vi "Home.vi"() -> ()   [LabVIEW 2020]
doc: "Fonction :\n\nCe modèle peut être intégré très facilement à un subpannel à l'aide des fonctions de la palette Code Template >> Dynamic VI and Subpanel de la VIBOX"
uses:
  System.Windows.Forms
  <vilib>/Platform/TimedLoop/XDataNode/timing_clust.ctl
  <vilib>/Platform/TimedLoop/XDataNode/nitl_modes.ctl
  <vilib>/Platform/TimedLoop/XDataNode/wakeup.ctl
  <vilib>/Platform/TimedLoop/XDataNode/XDataNode.xnode
  Program Files (x86)/National Instruments/LabVIEW 2020/examples/DataGrid for LabVIEW/DataGrid.lvlib
  <vilib>/Platform/TimedLoop/XDataNode/XDNodeRunTimeDep.lvlib
panel:
  in  "今日计划":refnum<k24>(container)
  out "Stop<user event>":refnum<user-event>
  in  "当前生产统计":refnum<k24>(container)
  in  "当前生产状态":refnum<k24>(container)
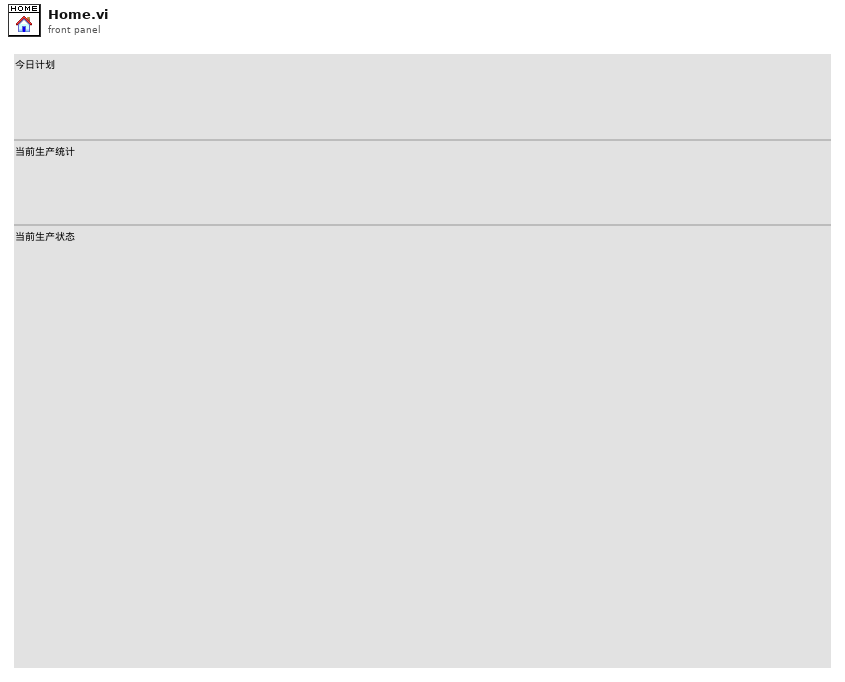
[diagram p1: front panel]
types:
  T1 = typedef "DataGrid.lvlib/GridColumn.lvclass/ColumnDefinition.ctl" = cluster{"name":string, "caption":string, "datatype":T2, "Params":string, "AutoSizeMode":i32, "FillWeight":sgl, "MinWidth":u32, "tooltip":string}
  T2 = typedef "DataGrid.lvlib/GridColumn.lvclass/ColumnType.ctl" = enum16{"string", "image", "check", "numeric", "timestamp", "button", "combo", "link"}
  T3 = typedef "XDNodeRunTimeDep.lvlib/timing_clust.ctl" = cluster{"Expected End [f-1]":u64, "Actual End [f-1]":u64, "Finished Late? [f-1]":bool, "Expected End [i-1]":u64, "Actual End [i-1]":u64, "Finished Late? [i-1]":bool, "Expected Start [i]":u64, "Actual Start [i]":u64, "Expected Start [f]":u64, "Actual Start [f]":u64, "Source Name":string, "Structure Name":string, "Period":i64, "Deadline":i64, "Offset":i64, "Start":i64, "Priority":i32, "Timeout":i32, "Mode":T4, "Wakeup Reason":T5, "Error":errorcluster, "Source Type":string, "Secondary Source Type":string, "Global End Time":u64, "Global Start Time":u64, "Frame Duration":u64, "Iteration Duration":u64, "Assigned CPU":i32, "I/O Scan Engine Mode":u32}
  T4 = typedef "XDNodeRunTimeDep.lvlib/nitl_modes.ctl" = enum32{"No Change", "Process missed periods, maintain original phase", "Discard missed periods, maintain original phase", "Process missed periods, ignore original phase", "Discard missed periods, ignore original phase"}
  T5 = typedef "XDNodeRunTimeDep.lvlib/wakeup.ctl" = enum32{"Normal", "Aborted", "Asynchronous wakeup", "Timing source error", "Timed loop error", "Timeout"}
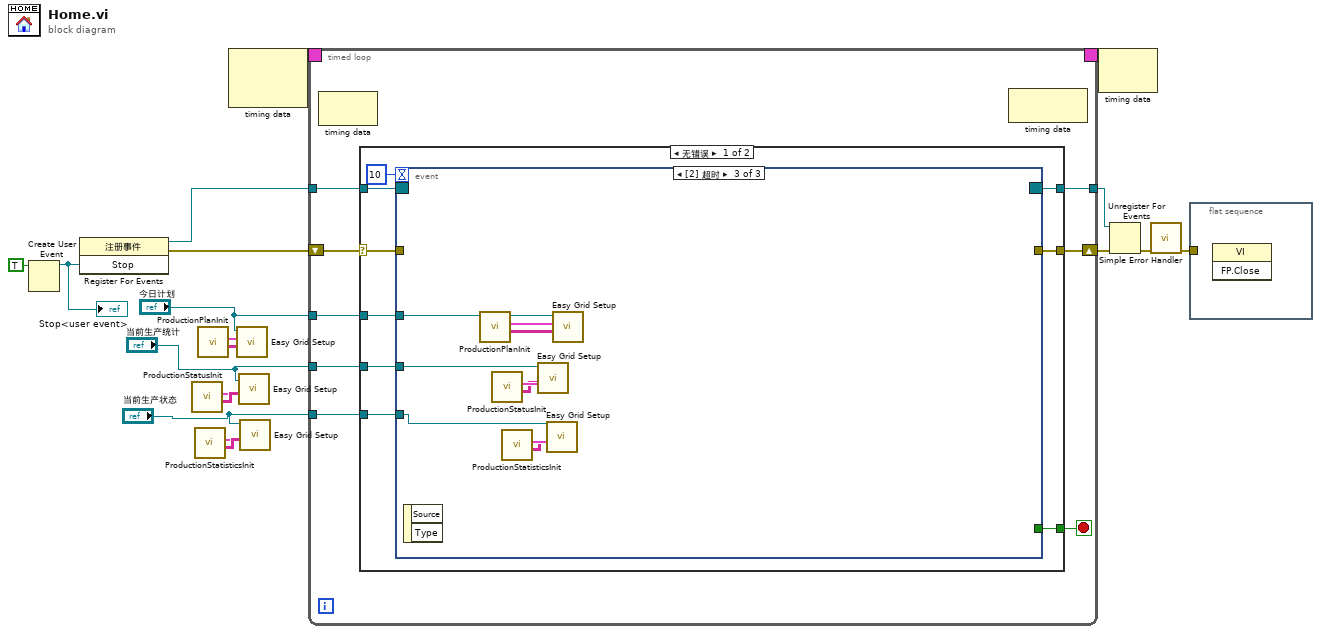
[diagram p0: block diagram]
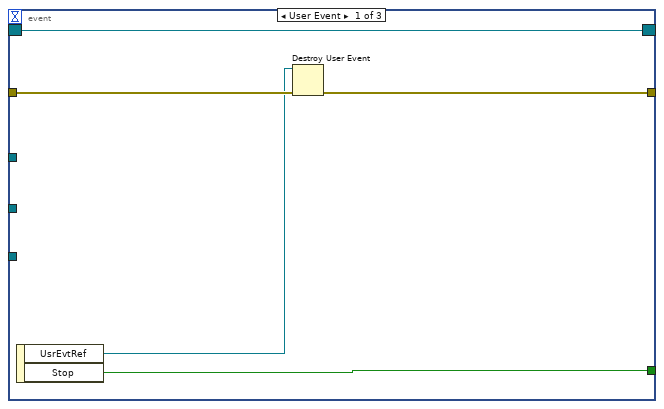
[diagram p2: hidden frame]
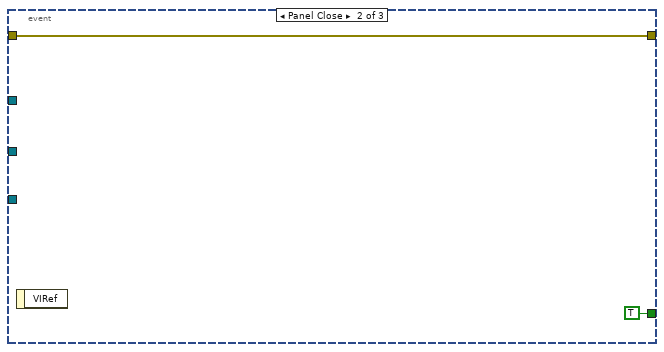
[diagram p3: hidden frame]
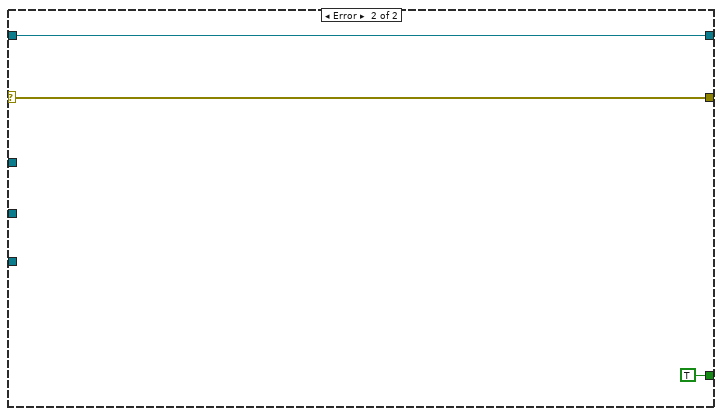
[diagram p4: hidden frame]
diagram:
  n1 = Create User Event(user event datatype=TRUE ("Stop")) -> (user event=w17:refnum<user-event>)  [unwired: 1 in, 1 out]
  "Stop<user event>" <- w17
  n2 = register-events(w17) -> (reference out=w16:refnum<event-registration>, error out=w12:errorcluster)  [unwired: 2 in]
  n3 = call "ProductionStatusInit.vi"() -> ("DataSource Data"=w6:string[][], "ColumnSetup"=w5:T1[])  [unwired: 10 in]
  n4 = call "ProductionStatisticsInit.vi"() -> ("DataSource Data"=w4:string[][], "ColumnSetup"=w3:T1[])  [unwired: 10 in]
  n5 = call "ProductionPlanInit.vi"() -> ("DataSource Data"=w11:string[][], "ColumnSetup"=w10:T1[])  [unwired: 10 in]
  n6 = node-c288() -> (w8:T3)  [unwired: 2 in]
  n7 = call <vilib>:"Easy Grid Setup.vi"("DataSource Data"=w11, "ColumnSetup"=w10, "DataGridView"="今日计划") -> ()  [unwired: 5 in, 4 out]
  n8 = call <vilib>:"Easy Grid Setup.vi"("DataSource Data"=w6, "ColumnSetup"=w5, "DataGridView"="当前生产统计") -> ()  [unwired: 5 in, 4 out]
  n9 = call <vilib>:"Easy Grid Setup.vi"("DataSource Data"=w4, "ColumnSetup"=w3, "DataGridView"="当前生产状态") -> ()  [unwired: 5 in, 4 out]
  n10 = timed-loop {
    tunnel: w16 -> [w25]
    tunnel: [w24] -> w19
    shift-right: [w26] -> w15
    shift-left: w12 -> [w27]
    tunnel: "今日计划" -> [w23]
    timing: w8 -> [_]
    timing-out: [_] -> w7
    tunnel: "当前生产统计" -> [w21]
    tunnel: "当前生产状态" -> [w20]
    stop <- w22 stop-if-true
    n11 = node-c288() -> ()  [unwired: 1 in, 1 out]
    n12 = case shown="无错误" w27 {
      selector: w27 -> [w35 w56]
      tunnel: [w34 w56] -> w26
      tunnel: [w36 TRUE] -> w22
      tunnel: w25 -> [w37 w55]
      tunnel: [w38 w55] -> w24
      tunnel: w23 -> [w33 _]
      tunnel: w21 -> [w31 _]
      tunnel: w20 -> [w30 _]
      frame No Error {
        n13 = event shown="[2] 超时" {
          selector: w37 -> [w43 _ _]
          dyn-events: [w43 _ _] -> w38
          timeout: 10 -> [_ _ _]
          tunnel: [w40 TRUE ("Stop") _] -> w36
          tunnel: w35 -> [w42 w44 _]
          tunnel: [w39 w44 _] -> w34
          tunnel: w33 -> [_ _ w52]
          tunnel: w31 -> [_ _ w49]
          tunnel: w30 -> [_ _ w46]
          event User Event {
            n14 = event-data() -> ("UsrEvtRef"=w41:refnum<user-event>, "Stop"=w40:bool)  [unwired: 1 out]
            n15 = Destroy User Event(user event=w41, error in=w42) -> (error out=w39:errorcluster)
          }
          event Panel Close {
            n16 = event-data() -> ()  [unwired: 2 out]
          }
          event Timeout {
            n17 = event-data() -> ()  [unwired: 3 out]
            n18 = call "ProductionPlanInit.vi"() -> ("DataSource Data"=w53:string[][], "ColumnSetup"=w54:T1[])  [unwired: 10 in]
            n19 = call "ProductionStatusInit.vi"() -> ("DataSource Data"=w50:string[][], "ColumnSetup"=w51:T1[])  [unwired: 10 in]
            n20 = call "ProductionStatisticsInit.vi"() -> ("DataSource Data"=w47:string[][], "ColumnSetup"=w48:T1[])  [unwired: 10 in]
            n21 = call <vilib>:"Easy Grid Setup.vi"("DataSource Data"=w50, "ColumnSetup"=w51, "DataGridView"=w49) -> ()  [unwired: 5 in, 4 out]
            n22 = call <vilib>:"Easy Grid Setup.vi"("DataSource Data"=w47, "ColumnSetup"=w48, "DataGridView"=w46) -> ()  [unwired: 5 in, 4 out]
            n23 = call <vilib>:"Easy Grid Setup.vi"("DataSource Data"=w53, "ColumnSetup"=w54, "DataGridView"=w52) -> ()  [unwired: 5 in, 4 out]
          }
        }
      }
      frame Error {
      }
    }
    n24 = node-c288() -> ()  [unwired: 1 in, 1 out]
  }
  n25 = node-c288(w7) -> ()  [unwired: 1 out]
  n26 = Unregister For Events(event registration refnum=w19, error in=w15) -> (error out=w18:errorcluster)
  n27 = call <vilib>:"Simple Error Handler.vi"("error in (no error)"=w18) -> ("error out"=w13:errorcluster)  [unwired: 1 in, 7 out]
  n28 = flat-sequence {
    tunnel: w13 -> [_]
    frame #0 {
      n29 = invoke class="VI" method="FP.Close"() -> ()  [unwired: 3 in, 3 out]
    }
  }
